vi "Saturation Enqueue.vi"(7 "Opposite End?":bool, 8 "error in (no error)":errorcluster, 9 "Data":variant, 10 "State":T1, 11 "Queue in":refnum<queue>) -> (0 "error out":errorcluster, 3 "Queue out":refnum<queue>)   [LabVIEW 2017, in "Saturation.lvclass"]
uses:
  Saturation.lvclass
  Type Defs/Saturation State.ctl
  Saturation.lvclass/Saturation.ctl
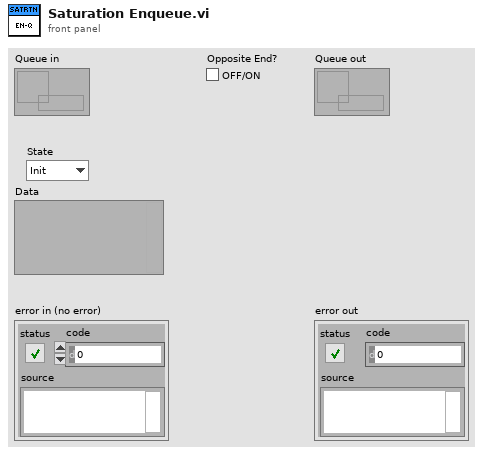
[diagram p1: front panel]
types:
  T1 = typedef "Saturation.lvclass/Saturation State.ctl" = enum16{"Init", "Update", "Go", "Stop", "Idle", "Error", "Shutdown"}
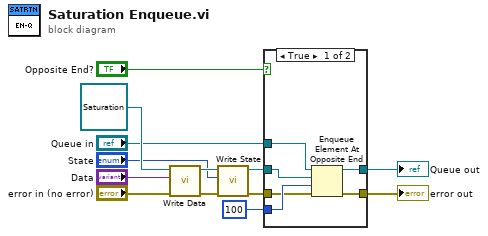
[diagram p0: block diagram]
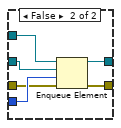
[diagram p2: hidden frame]
diagram:
  n1 = call "Write Data.vi"("error in (no error)"="error in (no error)", "Data"="Data", "Expansion in"=refnum<class "Saturation.lvclass"> refnum) -> ("error out"=w12:errorcluster, "Expansion out"=w13:refnum<class "Saturation.lvclass">)  [unwired: 7 in]
  n2 = call "Write State.vi"("error in (no error)"=w12, "State"="State", "Expansion in"=w13) -> ("error out"=w5:errorcluster, "Expansion out"=w8:refnum<class "Saturation.lvclass">)  [unwired: 7 in]
  n3 = case shown="True" "Opposite End?" {
    tunnel: [w19 w25] -> w4
    tunnel: "Queue in" -> [w18 w24]
    tunnel: 100 ("timeout in ms (-1)") -> [w17 w23]
    tunnel: w8 -> [w16 w22]
    tunnel: w5 -> [w15 w21]
    tunnel: [w14 w20] -> w3
    frame True {
      n4 = Enqueue Element At Opposite End(queue=w18, element=w16, timeout in ms (-1)=w17, error in (no error)=w15) -> (queue out=w19:refnum<queue>, error out=w14:errorcluster)  [unwired: 1 out]
    }
    frame False {
      n5 = Enqueue Element(queue=w24, element=w22, timeout in ms (-1)=w23, error in (no error)=w21) -> (queue out=w25:refnum<queue>, error out=w20:errorcluster)  [unwired: 1 out]
    }
  }
  "error out" <- w3
  "Queue out" <- w4
